vi "Ctrl.Ring.StyleFont.vi"(8 "error in (no error)":errorcluster, 10 "Font Info":T1, 11 "Ring Ref in":refnum<vi>) -> (0 "error out":errorcluster, 3 "Ring Ref out":refnum<vi>)   [LabVIEW 2017, in "JKI Simple Localization.lvlib"]
uses:
  API/JKI Simple Localization.lvlib
  Definitions/Private/Font Info -- Cluster.ctl
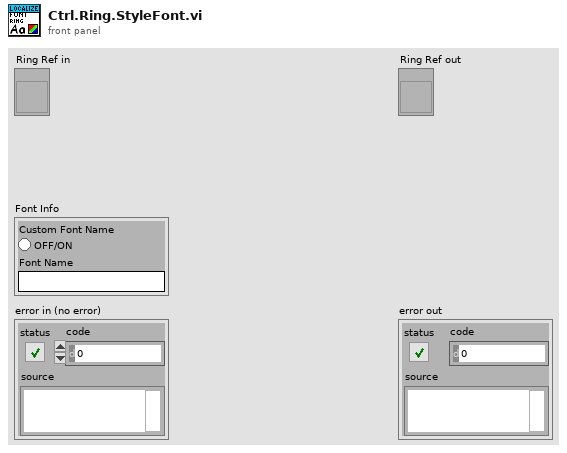
[diagram p1: front panel]
types:
  T1 = typedef "JKI Simple Localization.lvlib/Font Info -- Cluster.ctl" = cluster{"Custom Font Name":bool, "Font Name":string}
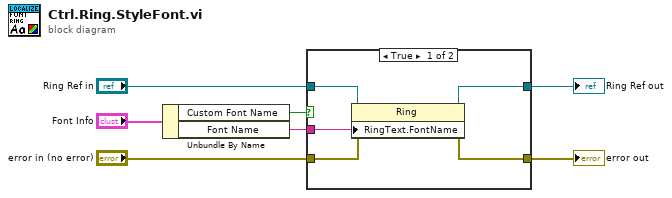
[diagram p0: block diagram]
diagram:
  n1 = Unbundle By Name("Font Info") -> ("Custom Font Name"=w6:bool, "Font Name"=w3:string)
  n2 = case shown="True" w6 {
    tunnel: [w9 w13] -> w5
    tunnel: "error in (no error)" -> [w10 w13]
    tunnel: w3 -> [w11 _]
    tunnel: "Ring Ref in" -> [w12 w14]
    tunnel: [w8 w14] -> w1
    frame True {
      n3 = property class="Ring"(reference=w12, error in=w10, "RingText.FontName"=w11) -> (reference out=w8:refnum<vi>, error out=w9:errorcluster)
    }
    frame False {
    }
  }
  "error out" <- w5
  "Ring Ref out" <- w1
